vi "display_for_debug.vi"(8 "error in (no error)":errorcluster, 11 "GenericTrajectory in":refnum<class "TrajectoryDL091126GenericVoxel.lvclass">) -> (0 "error out":errorcluster, 3 "GenericTrajectory out":refnum<class "TrajectoryDL091126GenericVoxel.lvclass">)   [LabVIEW 2010, in "TrajectoryDL091126GenericVoxel.lvclass"]
uses:
  TrajectoryDL091126GenericVoxel.lvclass
  common/enumerations/x_y_z_enumeration.ctl
  common/enumerations/functional_global_action_enum.ctl
panel:
  out "Intensity Graph":dbl[][](graph)
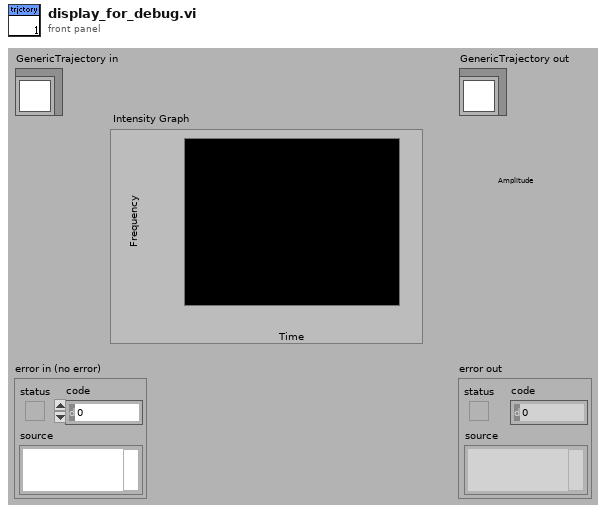
[diagram p1: front panel]
types:
  T1 = typedef "x_y_z_enumeration.ctl" = enum16{"x", "y", "z"}
  T2 = typedef "functional_global_action_enum.ctl" = enum16{"get", "set", "reset"}
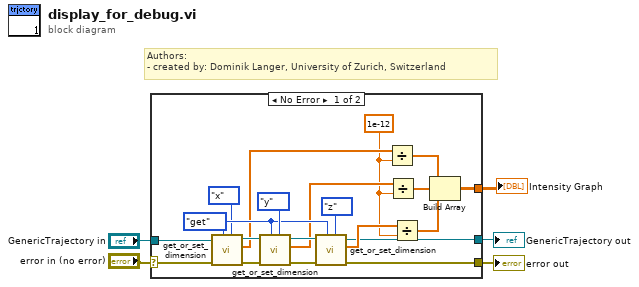
[diagram p0: block diagram]
diagram:
  # "Authors: \n- created by: Dominik Langer, University of Zurich, Switzerland"
  n1 = case shown="No Error" "error in (no error)" {
    selector: "error in (no error)" -> [w18 w27]
    tunnel: [w17 w27] -> w4
    tunnel: [w10 w26] -> w2
    tunnel: "GenericTrajectory in" -> [w11 w26]
    tunnel: [w6 _] -> w1
    frame No Error {
      w12 = dbl[unit] 1e-12 ("Numeric")
      w19 = functional_global_action_enum."get" ("action")
      n2 = call-dynamic "get_or_set_dimension.vi"("dimension"=x_y_z_enumeration."x", "action"=w19, "error in (no error)"=w18, "GenericTrajectory in"=w11) -> ("error out"=w22:errorcluster, "pixel values out (single dimension)"=w15:dbl[unit][], "GenericTrajectory out"=w21:refnum<class "TrajectoryDL091126GenericVoxel.lvclass">)  [unwired: 2 in, 3 out]
      n3 = call-dynamic "get_or_set_dimension.vi"("dimension"=x_y_z_enumeration."y", "action"=w19, "error in (no error)"=w22, "GenericTrajectory in"=w21) -> ("error out"=w23:errorcluster, "pixel values out (single dimension)"=w14:dbl[unit][], "GenericTrajectory out"=w20:refnum<class "TrajectoryDL091126GenericVoxel.lvclass">)  [unwired: 2 in, 3 out]
      n4 = call-dynamic "get_or_set_dimension.vi"("dimension"=x_y_z_enumeration."z", "action"=w19, "error in (no error)"=w23, "GenericTrajectory in"=w20) -> ("error out"=w17:errorcluster, "pixel values out (single dimension)"=w13:dbl[unit][], "GenericTrajectory out"=w10:refnum<class "TrajectoryDL091126GenericVoxel.lvclass">)  [unwired: 2 in, 3 out]
      n5 = Divide(x=w15, y=w12) -> (x/y=w9:dbl[])
      n6 = Divide(x=w14, y=w12) -> (x/y=w7:dbl[])
      n7 = Divide(x=w13, y=w12) -> (x/y=w8:dbl[])
      n8 = Build Array(w9, w7, w8) -> (w6:dbl[][])
    }
    frame Error {
    }
  }
  "error out" <- w4
  "GenericTrajectory out" <- w2
  "Intensity Graph" <- w1
